vi "Numato Relay ON OFF.vi"(8 "error in (no error)":errorcluster, 9 "Set Relay":bool, 10 "Relay Channel":u32 format="%.0x", 11 "VISA resource name":refnum<visa-resource-name>="COM4") -> (0 "error out":errorcluster, 1 "Success?":bool, 2 "Relay State":bool)   [LabVIEW 2025, in "Interface Functions.lvlib"]
doc: "Set a specific relay channel open/close (ON/OFF) on the Numato relay board. This function sends the \"relay on #\" or \"relay off #\" command to set the specified relay channel state, and subsequently sends the \"relay read #\" command to read back the current relay state to confirm the request was completed successfully."
uses:
  Interface Functions.lvlib
  <vilib>/regexp/Match Regular Expression.xnode
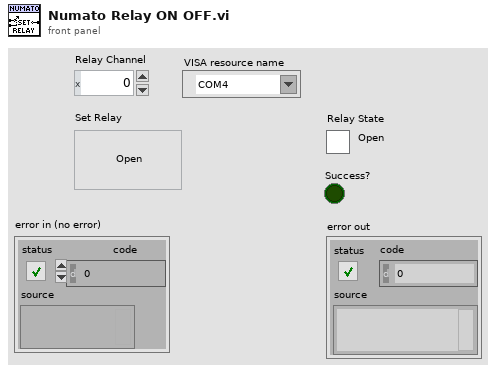
[diagram p1: front panel]
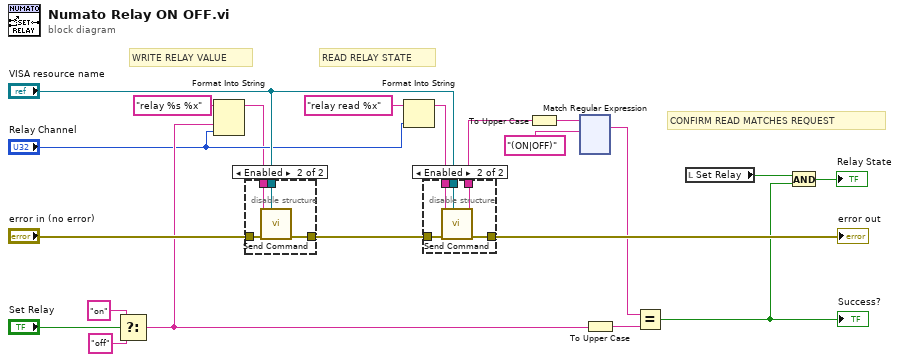
[diagram p0: block diagram]
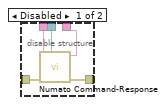
[diagram p2: hidden frame]
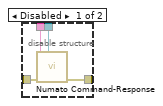
[diagram p3: hidden frame]
diagram:
  # "CONFIRM READ MATCHES REQUEST"
  # "READ RELAY STATE"
  # "WRITE RELAY VALUE"
  n1 = Select(t="on", s="Set Relay", f="off") -> (s? t:f=w12:string)
  n2 = Format Into String(format string="relay %s %x" ("write buffer"), w12, "Relay Channel") -> (resulting string=w2:string)  [unwired: 2 in, 1 out]
  n3 = disable-structure shown="Enabled" {
    disable-tunnel: "error in (no error)" -> [w25 w26]
    disable-tunnel: [w24 w27] -> w18
    disable-tunnel: "VISA resource name" -> [w23 w28]
    disable-tunnel: w2 -> [w22 w29]
    frame Disabled {
      n4 = call "Numato Command-Response.vi"("VISA resource name"=w23, "error in (no error)"=w25, "Command"=w22) -> ("error out"=w24:errorcluster)  [unwired: 7 in, 1 out]
    }
    frame Enabled {
      n5 = call "Send Command.vi"("error in (no error)"=w26, "Command"=w29, "VISA resource name"=w28) -> ("error out"=w27:errorcluster)  [unwired: 6 in, 2 out]
    }
  }
  n6 = Format Into String(format string="relay read %x" ("write buffer"), "Relay Channel") -> (resulting string=w3:string)  [unwired: 2 in, 1 out]
  n7 = disable-structure shown="Enabled" {
    disable-tunnel: w18 -> [w34 w39]
    disable-tunnel: [w33 w38] -> w17
    disable-tunnel: "VISA resource name" -> [w32 w37]
    disable-tunnel: w3 -> [w31 w36]
    disable-tunnel: [w30 w35] -> w1
    frame Disabled {
      n8 = call "Numato Command-Response.vi"("VISA resource name"=w32, "error in (no error)"=w34, "Command"=w31) -> ("error out"=w33:errorcluster, "Response"=w30:string)  [unwired: 7 in]
    }
    frame Enabled {
      n9 = call "Send Command.vi"("error in (no error)"=w39, "Command"=w36, "VISA resource name"=w37) -> ("error out"=w38:errorcluster, "Read Value"=w35:string)  [unwired: 6 in, 1 out]
    }
  }
  "error out" <- w17
  n10 = To Upper Case(1:w1) -> (0:w8:string)
  n11 = xnode "Match Regular Expression"("input string"=w8, "regular expression"="(ON|OFF)" ("format string")) -> ("whole match"=w7:string)  [unwired: 4 in, 4 out]
  n12 = To Upper Case(1:w12) -> (0:w11:string)
  n13 = Equal?(x=w7, y=w11) -> (x = y?=w5:bool)
  "Success?" <- w5
  n14 = local read "Set Relay"() -> (w6:bool)
  n15 = And(x=w6, y=w5) -> (x .and. y?=→"Relay State":bool)
